vi "benchmark-TagDB.vi"() -> (2 "read":dbl=2.8434400558471685e-05 format="%#_6f", 3 "write":dbl=2.78111743927002e-05 format="%#_6f")   [LabVIEW 2017]
uses:
  a6fc632b-2e92-436d-bf5a-00a40263cc33.vi
  5f513741-77c9-4122-96c3-2ffecd0507aa.vi
  TagDB/_Support/DataAccess/_NameCacher.vi
  TagDB/_Support/DataAccess/_datatypeChecker.vi
  TagDB/_Support/DataAccess/TagDB Ref to DVR.vi
  <vilib>/Utility/Data Type/Get Type Information.vi
  <vilib>/Utility/error.llb/Trim Whitespace.vi
  TagDB/_Support/Error/_[error50000]Invalid DB REF.vi
  TagDB/_Support/Error/_[error50002]Invalid DataType.vi
  <userlib>/_OpenG.lib/md5/md5.llb/MD5 Message Digest (Binary String)__ogtk.vi
  TagDB/TagDB(DEV).lvlib
panel:
  out "write 2":dbl=2.78111743927002e-05 caption="write" format="%#_6f"
  out "length":i32=1170
  out "outside":i32=499
  out "unit (s)":cluster{dbl[]}[](graph)=[{[4.010200500488281e-05, 2.005577087402344e-05, 3.0074119567871094e-05, 3.0078887939453124e-05, 3.0078887939453124e-05, 3.0078887939453124e-05, 2.0051002502441405e-05, 3.0078887939453124e-05, 3.0078887939453124e-05, 3.0078887939453124e-05, 3.0083656311035158e-05, 2.0847320556640624e-05, 2.9277801513671874e-05, 3.0078887939453124e-05, 3.0236244201660155e-05, 3.071784973144531e-05, 2.9430389404296874e-05, 2.002716064453125e-05, 2.9959678649902343e-05, 3.0078887939453124e-05, 3.0074119567871094e-05, 3.0231475830078124e-05, 2.0260810852050782e-05, 2.987384796142578e-05, 2.9926300048828124e-05, 3.0083656311035158e-05, 3.0069351196289064e-05, 3.0231475830078124e-05, 2.005577087402344e-05, 3.0074119567871094e-05, 2.9926300048828124e-05, 3.0078887939453124e-05, 3.0083656311035158e-05, 3.0078887939453124e-05, 2.0046234130859375e-05, 3.0088424682617188e-05, 3.0074119567871094e-05, 3.0078887939453124e-05, 3.0078887939453124e-05, 3.0078887939453124e-05, 2.0051002502441405e-05, 3.0078887939453124e-05, 3.0078887939453124e-05, 3.0078887939453124e-05, 3.0074119567871094e-05, 3.0078887939453124e-05, 2.005577087402344e-05, 3.0083656311035158e-05, 3.0078887939453124e-05, 3.0069351196289064e-05, 3.0083656311035158e-05, 3.0078887939453124e-05, 3.0078887939453124e-05, 2.0046234130859375e-05, 3.0083656311035158e-05, 3.0078887939453124e-05, 3.0078887939453124e-05, 3.0078887939453124e-05, 3.0083656311035158e-05, 2.0046234130859375e-05, 3.0078887939453124e-05, 3.0078887939453124e-05, 3.0083656311035158e-05, 3.0078887939453124e-05, 3.0069351196289064e-05, 2.006053924560547e-05, 3.0078887939453124e-05, 3.0078887939453124e-05, 3.0078887939453124e-05, 3.0074119567871094e-05, 2.005577087402344e-05, 3.0078887939453124e-05, 3.0078887939453124e-05, 3.0074119567871094e-05, 3.0078887939453124e-05, 3.0088424682617188e-05, 2.0046234130859375e-05, 3.0074119567871094e-05, 3.0078887939453124e-05, 3.0078887939453124e-05, 3.0083656311035158e-05, 3.0078887939453124e-05, 2.0046234130859375e-05, 3.0078887939453124e-05, 3.0083656311035158e-05, 3.0078887939453124e-05, 3.0078887939453124e-05, 3.0231475830078124e-05, 2.0051002502441405e-05, 2.9926300048828124e-05, 3.0078887939453124e-05, 3.0078887939453124e-05, 3.0074119567871094e-05, 2.005577087402344e-05, 3.0088424682617188e-05, 3.0074119567871094e-05, 3.0078887939453124e-05, 3.0069351196289064e-05, 2.005577087402344e-05, 3.0083656311035158e-05, 3.0078887939453124e-05, 3.0078887939453124e-05, 3.0074119567871094e-05, 3.0078887939453124e-05, 2.005577087402344e-05, 3.0069351196289064e-05, 3.0088424682617188e-05, 3.0074119567871094e-05, 3.0078887939453124e-05, 3.0078887939453124e-05, 3.0083656311035158e-05, 2.005577087402344e-05, 3.0069351196289064e-05, 3.0078887939453124e-05, 3.0083656311035158e-05, 3.0078887939453124e-05, 3.0078887939453124e-05, 2.0051002502441405e-05, 3.0078887939453124e-05, 3.0078887939453124e-05, 3.0078887939453124e-05, 3.0074119567871094e-05, 3.0078887939453124e-05, 2.005577087402344e-05, 3.0078887939453124e-05, 3.0083656311035158e-05, 3.0069351196289064e-05, 3.0078887939453124e-05, 3.024101257324219e-05, 2.0046234130859375e-05, 2.9931068420410158e-05, 3.0069351196289064e-05, 3.0088424682617188e-05, 3.0074119567871094e-05, 3.0231475830078124e-05, 3.0078887939453124e-05, 2.9931068420410158e-05, 3.0069351196289064e-05, 3.0078887939453124e-05, 2.005577087402344e-05, 2.0203590393066405e-05, 2.9931068420410158e-05, 3.0069351196289064e-05, 3.0083656311035158e-05, 3.0231475830078124e-05, 3.0078887939453124e-05, 2.005577087402344e-05, 2.9921531677246094e-05, 3.0078887939453124e-05, 3.0231475830078124e-05, 3.0078887939453124e-05, 3.0083656311035158e-05, 2.0046234130859375e-05, 2.9926300048828124e-05, 3.0078887939453124e-05, 3.0083656311035158e-05, 3.0069351196289064e-05, 2.02178955078125e-05, 3.0069351196289064e-05, 2.9931068420410158e-05, 3.0078887939453124e-05, 3.0074119567871094e-05, 3.0078887939453124e-05, 2.005577087402344e-05, 3.0078887939453124e-05, 3.0074119567871094e-05, 3.0078887939453124e-05, 3.0078887939453124e-05, 3.0078887939453124e-05, 3.0083656311035158e-05, 2.0046234130859375e-05, 3.0088424682617188e-05, 3.0069351196289064e-05, 3.0083656311035158e-05, 3.0078887939453124e-05, 3.0078887939453124e-05, 3.0074119567871094e-05, 2.005577087402344e-05, 3.0078887939453124e-05, 3.0078887939453124e-05, 3.0074119567871094e-05, 3.0078887939453124e-05, 3.0078887939453124e-05, 3.0078887939453124e-05, 2.005577087402344e-05, 3.0074119567871094e-05, 3.0078887939453124e-05, 3.0078887939453124e-05, 3.0083656311035158e-05, 3.0078887939453124e-05, 2.0046234130859375e-05, 3.0083656311035158e-05, 3.0078887939453124e-05, 3.0078887939453124e-05, 3.0078887939453124e-05, 3.0078887939453124e-05, 2.0051002502441405e-05, 3.0078887939453124e-05, 3.0231475830078124e-05, 3.0078887939453124e-05, 2.9931068420410158e-05, 3.0069351196289064e-05, 2.0847320556640624e-05, 2.944469451904297e-05, 3.0078887939453124e-05, 3.0069351196289064e-05, 2.9935836791992188e-05, 2.0203590393066405e-05, 3.071784973144531e-05, 2.9430389404296874e-05, 3.072261810302735e-05, 2.943992614746094e-05, 3.0078887939453124e-05, 2.005577087402344e-05, 3.0078887939453124e-05, 3.0074119567871094e-05, 3.0078887939453124e-05, 3.0078887939453124e-05, 3.0083656311035158e-05, 2.005577087402344e-05, 3.0069351196289064e-05, 3.072261810302735e-05, 2.943992614746094e-05, 3.0088424682617188e-05, 2.0046234130859375e-05, 3.0074119567871094e-05, 3.0078887939453124e-05, 3.0078887939453124e-05, 3.0078887939453124e-05, 3.0078887939453124e-05, 2.0051002502441405e-05, 3.0078887939453124e-05, 3.0078887939453124e-05, 3.0083656311035158e-05, 3.070831298828125e-05, 2.9449462890625e-05, 3.0078887939453124e-05, 2.0051002502441405e-05, 3.071784973144531e-05, 2.943992614746094e-05, 3.0074119567871094e-05, 3.0078887939453124e-05, 3.070354461669922e-05, 1.9431114196777344e-05, 3.0074119567871094e-05, 3.0078887939453124e-05, 3.0078887939453124e-05, 3.0112266540527343e-05, 3.005027770996094e-05, 2.005577087402344e-05, 3.0069351196289064e-05, 3.0078887939453124e-05, 3.0083656311035158e-05, 3.0078887939453124e-05, 3.0078887939453124e-05, 2.0051002502441405e-05, 3.0078887939453124e-05, 3.0078887939453124e-05, 3.0074119567871094e-05, 3.0083656311035158e-05, 3.0074119567871094e-05, 2.005577087402344e-05, 3.0078887939453124e-05, 3.0074119567871094e-05, 3.0078887939453124e-05, 3.0078887939453124e-05, 3.072261810302735e-05, 1.941680908203125e-05, 3.070831298828125e-05, 2.943992614746094e-05, 3.0083656311035158e-05, 3.0078887939453124e-05, 3.0078887939453124e-05, 2.0046234130859375e-05, 3.0083656311035158e-05, 3.0078887939453124e-05, 3.0078887939453124e-05, 3.0078887939453124e-05, 2.0051002502441405e-05, 3.071784973144531e-05, 2.943992614746094e-05, 3.0078887939453124e-05, 3.0083656311035158e-05, 3.0078887939453124e-05, 2.0046234130859375e-05, 3.0083656311035158e-05, 3.0078887939453124e-05, 3.0069351196289064e-05, 2.9935836791992188e-05, 3.0074119567871094e-05, 3.0078887939453124e-05, 2.0051002502441405e-05, 3.0231475830078124e-05, 3.0078887939453124e-05, 2.9926300048828124e-05, 3.0088424682617188e-05, 3.0074119567871094e-05, 3.0078887939453124e-05, 2.020835876464844e-05, 3.0069351196289064e-05, 2.9931068420410158e-05, 3.0078887939453124e-05, 3.0078887939453124e-05, 3.0074119567871094e-05, 3.0078887939453124e-05, 3.0078887939453124e-05, 2.0051002502441405e-05, 3.0078887939453124e-05, 3.0078887939453124e-05, 3.0078887939453124e-05, 3.0083656311035158e-05, 3.0078887939453124e-05, 3.0069351196289064e-05, 2.005577087402344e-05, 3.0083656311035158e-05, 3.0078887939453124e-05, 3.0078887939453124e-05, 3.0074119567871094e-05, 3.0078887939453124e-05, 2.005577087402344e-05, 3.0078887939453124e-05, 3.0074119567871094e-05, 3.0078887939453124e-05, 3.0078887939453124e-05, 3.0078887939453124e-05, 2.0051002502441405e-05, 3.0078887939453124e-05, 3.024101257324219e-05, 3.0069351196289064e-05, 2.9931068420410158e-05, 2.0046234130859375e-05, 3.024101257324219e-05, 3.0112266540527343e-05, 2.9888153076171875e-05, 3.0112266540527343e-05, 3.0045509338378905e-05, 3.0078887939453124e-05, 2.0051002502441405e-05, 3.0078887939453124e-05, 3.0231475830078124e-05, 3.0078887939453124e-05, 2.9931068420410158e-05, 3.0069351196289064e-05, 2.0847320556640624e-05, 2.943992614746094e-05, 3.072261810302735e-05, 2.9430389404296874e-05, 3.0083656311035158e-05, 3.0078887939453124e-05, 2.005577087402344e-05, 3.0078887939453124e-05, 3.0074119567871094e-05, 2.9935836791992188e-05, 3.0221939086914064e-05, 3.0078887939453124e-05, 2.005577087402344e-05, 3.071308135986328e-05, 2.943992614746094e-05, 3.0112266540527343e-05, 3.005027770996094e-05, 3.071784973144531e-05, 2.943992614746094e-05, 2.0046234130859375e-05, 3.0083656311035158e-05, 2.9926300048828124e-05, 3.0231475830078124e-05, 3.0078887939453124e-05, 2.0051002502441405e-05, 3.0078887939453124e-05, 3.071784973144531e-05, 2.943992614746094e-05, 3.0074119567871094e-05, 3.0078887939453124e-05, 2.0694732666015624e-05, 2.9435157775878905e-05, 3.0078887939453124e-05, 3.0088424682617188e-05, 3.0074119567871094e-05, 3.0078887939453124e-05, 2.0046234130859375e-05, 3.0078887939453124e-05, 3.0083656311035158e-05, 3.0078887939453124e-05, 3.0088424682617188e-05, 2.0046234130859375e-05, 3.0074119567871094e-05, 3.0078887939453124e-05, 3.0078887939453124e-05, 3.0078887939453124e-05, 3.0083656311035158e-05, 2.0046234130859375e-05, 3.0078887939453124e-05, 3.0078887939453124e-05, 3.0074119567871094e-05, 3.0078887939453124e-05, 3.0078887939453124e-05, 2.005577087402344e-05, 3.0083656311035158e-05, 3.0078887939453124e-05, 3.0088424682617188e-05, 3.006458282470703e-05, 3.0078887939453124e-05, 2.005577087402344e-05, 3.0074119567871094e-05, 3.0078887939453124e-05, 3.0078887939453124e-05, 3.0078887939453124e-05, 3.0083656311035158e-05, 3.0078887939453124e-05, 2.0046234130859375e-05, 3.0078887939453124e-05, 3.0083656311035158e-05, 3.0078887939453124e-05, 3.0078887939453124e-05, 3.0074119567871094e-05, 3.0078887939453124e-05, 2.0694732666015624e-05, 2.943992614746094e-05, 3.0078887939453124e-05, 3.0083656311035158e-05, 3.070831298828125e-05, 2.943992614746094e-05, 2.005577087402344e-05, 2.9931068420410158e-05, 3.0069351196289064e-05, 3.0231475830078124e-05, 3.0083656311035158e-05, 3.009319305419922e-05, 3.005504608154297e-05, 1.99127197265625e-05, 3.0226707458496094e-05, 3.0078887939453124e-05, 3.0078887939453124e-05, 3.072261810302735e-05, 2.928733825683594e-05, 2.0046234130859375e-05, 3.0078887939453124e-05, 3.0236244201660155e-05, 3.0069351196289064e-05, 3.025054931640625e-05, 2.9764175415039063e-05, 2.0051002502441405e-05, 3.0069351196289064e-05, 3.0088424682617188e-05, 3.0226707458496094e-05, 3.0078887939453124e-05, 2.9926300048828124e-05, 2.0051002502441405e-05, 3.0078887939453124e-05, 3.0078887939453124e-05, 3.0078887939453124e-05, 3.0231475830078124e-05, 2.9931068420410158e-05, 2.0046234130859375e-05, 3.0078887939453124e-05, 3.0083656311035158e-05, 3.0231475830078124e-05, 2.9926300048828124e-05, 2.0046234130859375e-05, 3.0083656311035158e-05, 3.0078887939453124e-05, 3.0078887939453124e-05, 3.0231475830078124e-05, 2.9921531677246094e-05, 3.0088424682617188e-05, 2.0046234130859375e-05, 3.0074119567871094e-05, 3.0078887939453124e-05, 3.0078887939453124e-05, 3.0078887939453124e-05, 3.0083656311035158e-05, 2.005577087402344e-05, 3.0069351196289064e-05, 3.0083656311035158e-05, 3.0078887939453124e-05, 3.0078887939453124e-05, 3.0078887939453124e-05, 2.0051002502441405e-05, 3.0078887939453124e-05, 3.0231475830078124e-05, 3.0078887939453124e-05, 2.9931068420410158e-05, 3.0078887939453124e-05, 2.0046234130859375e-05, 3.0078887939453124e-05, 3.0231475830078124e-05, 3.0083656311035158e-05, 2.9926300048828124e-05, 3.0074119567871094e-05, 2.0847320556640624e-05, 2.9430389404296874e-05, 2.9926300048828124e-05, 3.0083656311035158e-05, 3.0088424682617188e-05, 3.0069351196289064e-05, 2.0051002502441405e-05, 3.0078887939453124e-05, 3.0078887939453124e-05, 3.0078887939453124e-05, 3.0078887939453124e-05]}, ...(2 in all)]
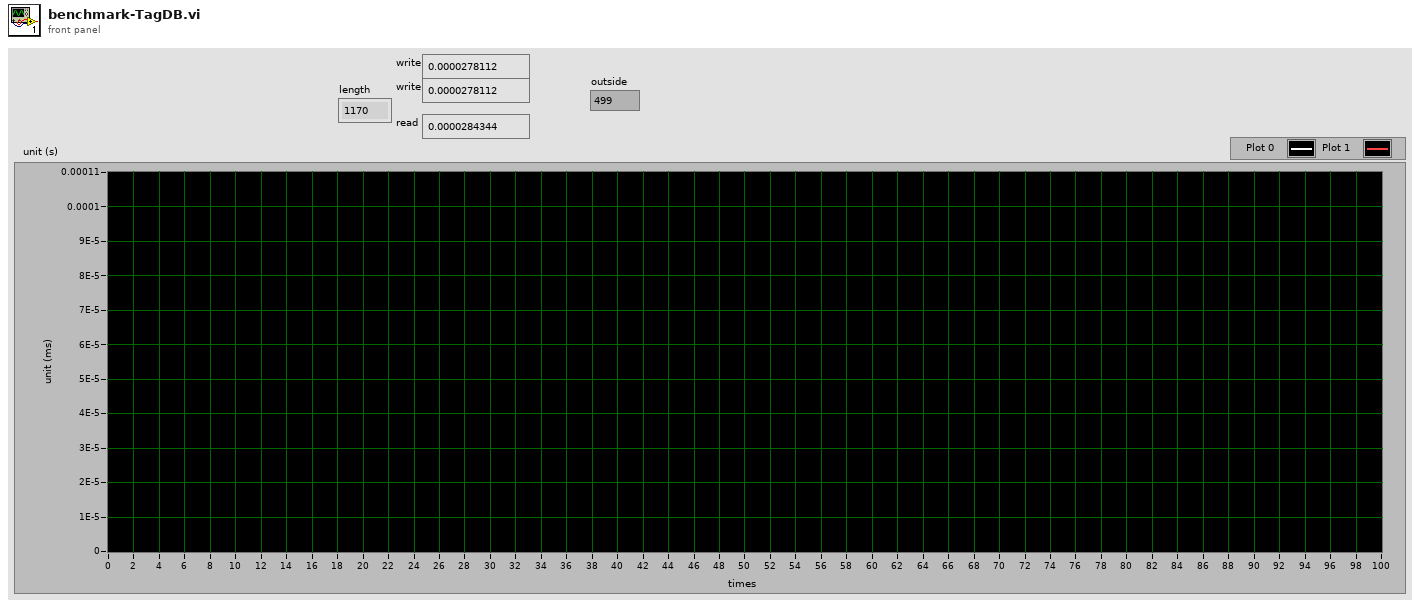
[diagram p1: front panel]
types:
  T1 = cluster{"error constant":errorcluster, "error constant 2":errorcluster, "error constant 3":errorcluster, "error constant 4":errorcluster, "error constant 5":errorcluster, "error constant 6":errorcluster, "error constant 7":errorcluster, "error constant 8":errorcluster, "error constant 9":errorcluster, "error constant 10":errorcluster, "error constant 11":errorcluster, "error constant 12":errorcluster, "error constant 13":errorcluster, "error constant 14":errorcluster, "error constant 15":errorcluster, "error constant 16":errorcluster, "error constant 17":errorcluster, "error constant 18":errorcluster, "error constant 19":errorcluster, "error constant 20":errorcluster, "error constant 21":errorcluster, "error constant 22":errorcluster, "error constant 23":errorcluster, "error constant 24":errorcluster, "error constant 25":errorcluster, "error constant 26":errorcluster, "error constant 27":errorcluster, "error constant 28":errorcluster, "error constant 29":errorcluster, "error constant 30":errorcluster, "error constant 31":errorcluster, "error constant 32":errorcluster, "error constant 33":errorcluster, "error constant 34":errorcluster, "error constant 35":errorcluster, "error constant 36":errorcluster, "error constant 37":errorcluster, "error constant 38":errorcluster, "error constant 39":errorcluster, "error constant 40":errorcluster, "error constant 41":errorcluster, "error constant 42":errorcluster, "error constant 43":errorcluster, "error constant 44":errorcluster, "error constant 45":errorcluster, "error constant 46":errorcluster, "error constant 47":errorcluster, "error constant 48":errorcluster, "error constant 49":errorcluster, "error constant 50":errorcluster, "error constant 51":errorcluster, "error constant 52":errorcluster, "error constant 53":errorcluster, "error constant 54":errorcluster, "error constant 55":errorcluster, "error constant 56":errorcluster, "error constant 57":errorcluster, "error constant 58":errorcluster, "error constant 59":errorcluster, "error constant 60":errorcluster, "error constant 61":errorcluster, "error constant 62":errorcluster, "error constant 63":errorcluster, "error constant 64":errorcluster, "error constant 65":errorcluster, cluster{"error constant":errorcluster, "error constant 2":errorcluster, "error constant 3":errorcluster, "error constant 4":errorcluster, "error constant 5":errorcluster, "error constant 6":errorcluster, "error constant 7":errorcluster, "error constant 8":errorcluster, "error constant 9":errorcluster, "error constant 10":errorcluster, "error constant 11":errorcluster, "error constant 12":errorcluster, "error constant 13":errorcluster, "error constant 14":errorcluster, "error constant 15":errorcluster, "error constant 16":errorcluster, "error constant 17":errorcluster, "error constant 18":errorcluster, "error constant 19":errorcluster, "error constant 20":errorcluster, "error constant 21":errorcluster, "error constant 22":errorcluster, "error constant 23":errorcluster, "error constant 24":errorcluster, "error constant 25":errorcluster, "error constant 26":errorcluster, "error constant 27":errorcluster, "error constant 28":errorcluster, "error constant 29":errorcluster, "error constant 30":errorcluster, "error constant 31":errorcluster, "error constant 32":errorcluster, "error constant 33":errorcluster, "error constant 34":errorcluster, "error constant 35":errorcluster, "error constant 36":errorcluster, "error constant 37":errorcluster, "error constant 38":errorcluster, "error constant 39":errorcluster, "error constant 40":errorcluster, "error constant 41":errorcluster, "error constant 42":errorcluster, "error constant 43":errorcluster, "error constant 44":errorcluster, "error constant 45":errorcluster, "error constant 46":errorcluster, "error constant 47":errorcluster, "error constant 48":errorcluster, "error constant 49":errorcluster, "error constant 50":errorcluster, "error constant 51":errorcluster, "error constant 52":errorcluster, "error constant 53":errorcluster, "error constant 54":errorcluster, "error constant 55":errorcluster, "error constant 56":errorcluster, "error constant 57":errorcluster, "error constant 58":errorcluster, "error constant 59":errorcluster, "error constant 60":errorcluster, "error constant 61":errorcluster, "error constant 62":errorcluster, "error constant 63":errorcluster, "error constant 64":errorcluster, "error constant 65":errorcluster}}
  T2 = typedef "TagDB(DEV).lvlib/TagContainer.ctl" = refnum<k1>
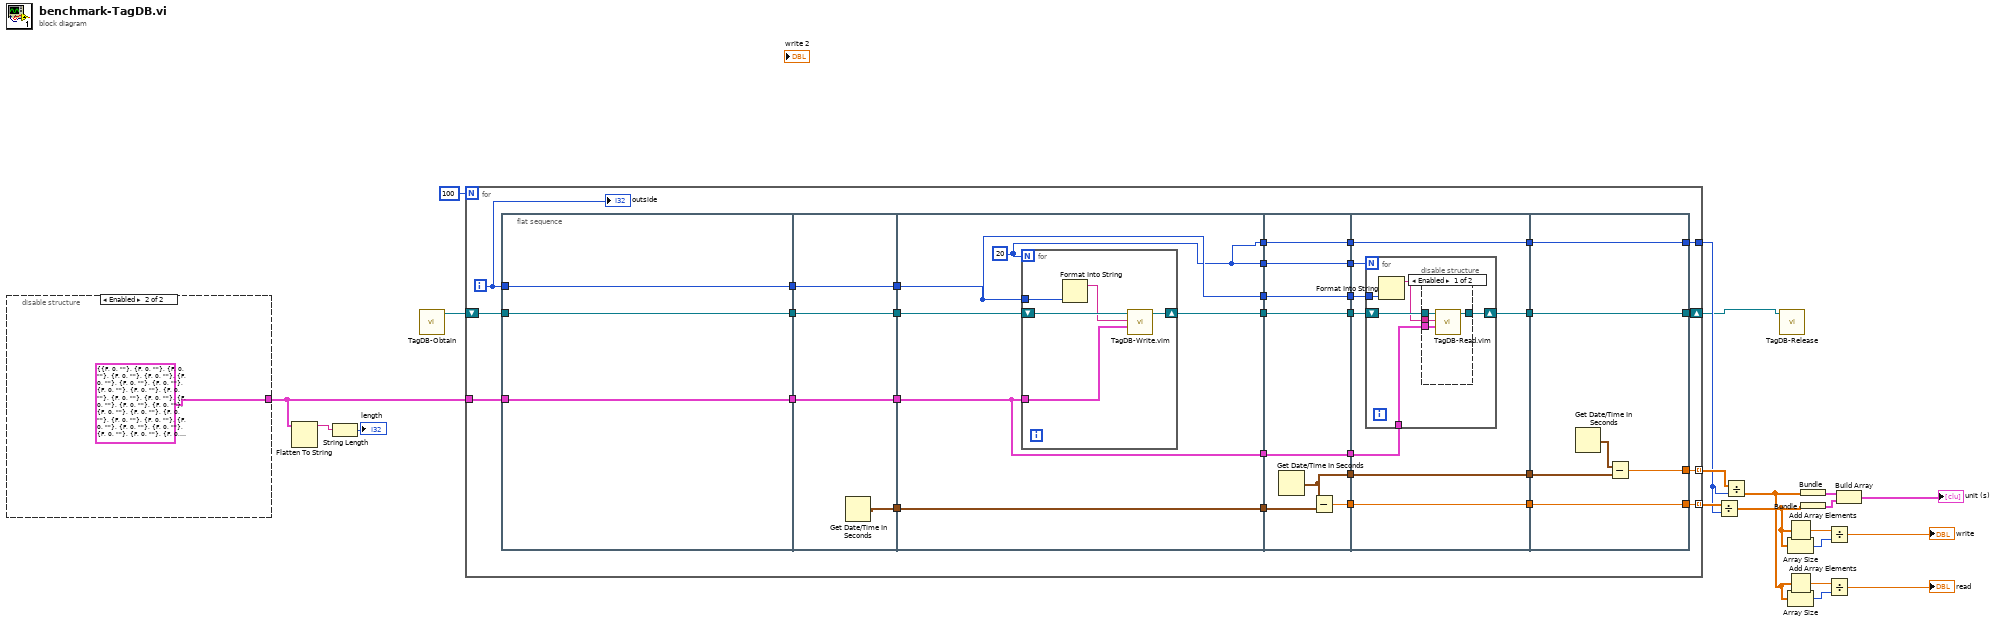
[diagram p0: block diagram]
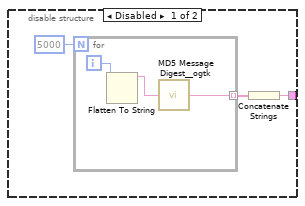
[diagram p2: hidden frame]
diagram:
  n1 = disable-structure shown="Enabled" {
    disable-tunnel: [w21 T1 {"error constant"={"status"=FALSE, "code"=0, "source"=""}, "error constant 2"={"status"=FALSE, "code"=0, "source"=""}, "error constant 3"={"status"=FALSE, "code"=0, "source"=""}, "error constant 4"={"status"=FALSE, "code"=0, "source"=""}, "error constant 5"={"status"=FALSE, "code"=0, "source"=""}, "error constant 6"={"status"=FALSE, "code"=0, "source"=""}, "error constant 7"={"status"=FALSE, "code"=0, "source"=""}, "error constant 8"={"status"=FALSE, "code"=0, "source"=""}, "error constant 9"={"status"=FALSE, "code"=0, "source"=""}, "error constant 10"={"status"=FALSE, "code"=0, "source"=""}, "error constant 11"={"status"=FALSE, "code"=0, "source"=""}, "error constant 12"={"status"=FALSE, "code"=0, "source"=""}, "error constant 13"={"status"=FALSE, "code"=0, "source"=""}, "error constant 14"={"status"=FALSE, "code"=0, "source"=""}, "error constant 15"={"status"=FALSE, "code"=0, "source"=""}, "error constant 16"={"status"=FALSE, "code"=0, "source"=""}, "error constant 17"={"status"=FALSE, "code"=0, "source"=""}, "error constant 18"={"status"=FALSE, "code"=0, "source"=""}, "error constant 19"={"status"=FALSE, "code"=0, "source"=""}, "error constant 20"={"status"=FALSE, "code"=0, "source"=""}, "error constant 21"={"status"=FALSE, "code"=0, "source"=""}, "error constant 22"={"status"=FALSE, "code"=0, "source"=""}, "error constant 23"={"status"=FALSE, "code"=0, "source"=""}, "error constant 24"={"status"=FALSE, "code"=0, "source"=""}, "error constant 25"={"status"=FALSE, "code"=0, "source"=""}, "error constant 26"={"status"=FALSE, "code"=0, "source"=""}, "error constant 27"={"status"=FALSE, "code"=0, "source"=""}, "error constant 28"={"status"=FALSE, "code"=0, "source"=""}, "error constant 29"={"status"=FALSE, "code"=0, "source"=""}, "error constant 30"={"status"=FALSE, "code"=0, "source"=""}, "error constant 31"={"status"=FALSE, "code"=0, "source"=""}, "error constant 32"={"status"=FALSE, "code"=0, "source"=""}, "error constant 33"={"status"=FALSE, "code"=0, "source"=""}, "error constant 34"={"status"=FALSE, "code"=0, "source"=""}, "error constant 35"={"status"=FALSE, "code"=0, "source"=""}, "error constant 36"={"status"=FALSE, "code"=0, "source"=""}, "error constant 37"={"status"=FALSE, "code"=0, "source"=""}, "error constant 38"={"status"=FALSE, "code"=0, "source"=""}, "error constant 39"={"status"=FALSE, "code"=0, "source"=""}, "error constant 40"={"status"=FALSE, "code"=0, "source"=""}, "error constant 41"={"status"=FALSE, "code"=0, "source"=""}, "error constant 42"={"status"=FALSE, "code"=0, "source"=""}, "error constant 43"={"status"=FALSE, "code"=0, "source"=""}, "error constant 44"={"status"=FALSE, "code"=0, "source"=""}, "error constant 45"={"status"=FALSE, "code"=0, "source"=""}, "error constant 46"={"status"=FALSE, "code"=0, "source"=""}, "error constant 47"={"status"=FALSE, "code"=0, "source"=""}, "error constant 48"={"status"=FALSE, "code"=0, "source"=""}, "error constant 49"={"status"=FALSE, "code"=0, "source"=""}, "error constant 50"={"status"=FALSE, "code"=0, "source"=""}, "error constant 51"={"status"=FALSE, "code"=0, "source"=""}, "error constant 52"={"status"=FALSE, "code"=0, "source"=""}, "error constant 53"={"status"=FALSE, "code"=0, "source"=""}, "error constant 54"={"status"=FALSE, "code"=0, "source"=""}, "error constant 55"={"status"=FALSE, "code"=0, "source"=""}, "error constant 56"={"status"=FALSE, "code"=0, "source"=""}, "error constant 57"={"status"=FALSE, "code"=0, "source"=""}, "error constant 58"={"status"=FALSE, "code"=0, "source"=""}, "error constant 59"={"status"=FALSE, "code"=0, "source"=""}, "error constant 60"={"status"=FALSE, "code"=0, "source"=""}, "error constant 61"={"status"=FALSE, "code"=0, "source"=""}, "error constant 62"={"status"=FALSE, "code"=0, "source"=""}, "error constant 63"={"status"=FALSE, "code"=0, "source"=""}, "error constant 64"={"status"=FALSE, "code"=0, "source"=""}, "error constant 65"={"status"=FALSE, "code"=0, "source"=""}, {"error constant"={"status"=FALSE, "code"=0, "source"=""}, "error constant 2"={"status"=FALSE, "code"=0, "source"=""}, "error constant 3"={"status"=FALSE, "code"=0, "source"=""}, "error constant 4"={"status"=FALSE, "code"=0, "source"=""}, "error constant 5"={"status"=FALSE, "code"=0, "source"=""}, "error constant 6"={"status"=FALSE, "code"=0, "source"=""}, "error constant 7"={"status"=FALSE, "code"=0, "source"=""}, "error constant 8"={"status"=FALSE, "code"=0, "source"=""}, "error constant 9"={"status"=FALSE, "code"=0, "source"=""}, "error constant 10"={"status"=FALSE, "code"=0, "source"=""}, "error constant 11"={"status"=FALSE, "code"=0, "source"=""}, "error constant 12"={"status"=FALSE, "code"=0, "source"=""}, "error constant 13"={"status"=FALSE, "code"=0, "source"=""}, "error constant 14"={"status"=FALSE, "code"=0, "source"=""}, "error constant 15"={"status"=FALSE, "code"=0, "source"=""}, "error constant 16"={"status"=FALSE, "code"=0, "source"=""}, "error constant 17"={"status"=FALSE, "code"=0, "source"=""}, "error constant 18"={"status"=FALSE, "code"=0, "source"=""}, "error constant 19"={"status"=FALSE, "code"=0, "source"=""}, "error constant 20"={"status"=FALSE, "code"=0, "source"=""}, "error constant 21"={"status"=FALSE, "code"=0, "source"=""}, "error constant 22"={"status"=FALSE, "code"=0, "source"=""}, "error constant 23"={"status"=FALSE, "code"=0, "source"=""}, "error constant 24"={"status"=FALSE, "code"=0, "source"=""}, "error constant 25"={"status"=FALSE, "code"=0, "source"=""}, "error constant 26"={"status"=FALSE, "code"=0, "source"=""}, "error constant 27"={"status"=FALSE, "code"=0, "source"=""}, "error constant 28"={"status"=FALSE, "code"=0, "source"=""}, "error constant 29"={"status"=FALSE, "code"=0, "source"=""}, "error constant 30"={"status"=FALSE, "code"=0, "source"=""}, "error constant 31"={"status"=FALSE, "code"=0, "source"=""}, "error constant 32"={"status"=FALSE, "code"=0, "source"=""}, "error constant 33"={"status"=FALSE, "code"=0, "source"=""}, "error constant 34"={"status"=FALSE, "code"=0, "source"=""}, "error constant 35"={"status"=FALSE, "code"=0, "source"=""}, "error constant 36"={"status"=FALSE, "code"=0, "source"=""}, "error constant 37"={"status"=FALSE, "code"=0, "source"=""}, "error constant 38"={"status"=FALSE, "code"=0, "source"=""}, "error constant 39"={"status"=FALSE, "code"=0, "source"=""}, "error constant 40"={"status"=FALSE, "code"=0, "source"=""}, "error constant 41"={"status"=FALSE, "code"=0, "source"=""}, "error constant 42"={"status"=FALSE, "code"=0, "source"=""}, "error constant 43"={"status"=FALSE, "code"=0, "source"=""}, "error constant 44"={"status"=FALSE, "code"=0, "source"=""}, "error constant 45"={"status"=FALSE, "code"=0, "source"=""}, "error constant 46"={"status"=FALSE, "code"=0, "source"=""}, "error constant 47"={"status"=FALSE, "code"=0, "source"=""}, "error constant 48"={"status"=FALSE, "code"=0, "source"=""}, "error constant 49"={"status"=FALSE, "code"=0, "source"=""}, "error constant 50"={"status"=FALSE, "code"=0, "source"=""}, "error constant 51"={"status"=FALSE, "code"=0, "source"=""}, "error constant 52"={"status"=FALSE, "code"=0, "source"=""}, "error constant 53"={"status"=FALSE, "code"=0, "source"=""}, "error constant 54"={"status"=FALSE, "code"=0, "source"=""}, "error constant 55"={"status"=FALSE, "code"=0, "source"=""}, "error constant 56"={"status"=FALSE, "code"=0, "source"=""}, "error constant 57"={"status"=FALSE, "code"=0, "source"=""}, "error constant 58"={"status"=FALSE, "code"=0, "source"=""}, "error constant 59"={"status"=FALSE, "code"=0, "source"=""}, "error constant 60"={"status"=FALSE, "code"=0, "source"=""}, "error constant 61"={"status"=FALSE, "code"=0, "source"=""}, "error constant 62"={"status"=FALSE, "code"=0, "source"=""}, "error constant 63"={"status"=FALSE, "code"=0, "source"=""}, "error constant 64"={"status"=FALSE, "code"=0, "source"=""}, "error constant 65"={"status"=FALSE, "code"=0, "source"=""}}}] -> w17
    frame Disabled {
      n2 = for {
        N: 5000 -> [_]
        tunnel: [w26] -> w23 mode=indexing
        i -> [w25]
        n3 = Flatten To String(anything=w25) -> (data string=w24:string)  [unwired: 3 in, 2 out]
        n4 = call-poly <userlib>:"MD5 Message Digest__ogtk.vi"("Message"=w24) -> ("MD5 Message Digest"=w26:string)
      }
      n5 = Concatenate Strings(w23) -> (w21:string)
    }
    frame Enabled {
    }
  }
  n6 = Flatten To String(anything=w17) -> (data string=w16:string)  [unwired: 3 in, 2 out]
  n7 = String Length(string=w16) -> (length=→"length":i32)
  n8 = call "TagDB-Obtain.vi"() -> ("TagContainer"=w2:T2)  [unwired: 5 in, 2 out]
  n9 = for {
    N: 100 -> [_]
    tunnel: [w56] -> w20 mode=indexing
    tunnel: [w55] -> w3
    tunnel: w17 -> [w42]
    shift-right: [w40] -> w1
    shift-left: w2 -> [w41]
    tunnel: [w35] -> w4 mode=indexing
    i -> [w53]
    n10 = flat-sequence {
      tunnel: w53 -> [w61]
      tunnel: [w59] -> w47
      tunnel: [w60] -> w45
      tunnel: [w61] -> w44
      tunnel: w42 -> [w60]
      tunnel: w41 -> [w59]
      tunnel: [w65] -> w58
      tunnel: [w64] -> w48
      tunnel: w47 -> [w64]
      tunnel: [w63] -> w46
      tunnel: w45 -> [w63]
      tunnel: w44 -> [w62]
      tunnel: [w62] -> w43
      tunnel: w58 -> [w71]
      tunnel: [w71] -> w57
      tunnel: [w67] -> w54
      tunnel: [w69] -> w49
      tunnel: w48 -> [w70]
      tunnel: w46 -> [w66]
      tunnel: w43 -> [w68]
      tunnel: [w67] -> w33
      tunnel: [w68] -> w30
      tunnel: [w66] -> w29
      tunnel: w57 -> [w81]
      tunnel: w54 -> [w83]
      tunnel: [w84] -> w52
      tunnel: [w83] -> w51
      tunnel: [w82] -> w50
      tunnel: w49 -> [w82]
      tunnel: [w77] -> w37
      tunnel: w33 -> [w80]
      tunnel: [w80] -> w32
      tunnel: [w79] -> w31
      tunnel: w30 -> [w79]
      tunnel: w29 -> [w78]
      tunnel: [w78] -> w28
      tunnel: w52 -> [w92]
      tunnel: w51 -> [w91]
      tunnel: w50 -> [w89]
      tunnel: [w92] -> w39
      tunnel: [w91] -> w38
      tunnel: w37 -> [w90]
      tunnel: [w90] -> w36
      tunnel: [w88] -> w34
      tunnel: w32 -> [w87]
      tunnel: w31 -> [w86]
      tunnel: w28 -> [w85]
      tunnel: [w106] -> w40
      tunnel: [w107] -> w55
      tunnel: [w108] -> w56
      tunnel: w39 -> [w108]
      tunnel: w38 -> [w107]
      tunnel: w36 -> [w104]
      tunnel: [w103] -> w35
      tunnel: w34 -> [w106]
      frame #0 {
      }
      frame #1 {
        n11 = Get Date/Time In Seconds() -> (seconds since 1Jan1904=w65:timestamp)
      }
      frame #2 {
        w67 = 20
        n12 = for {
          N: w67 -> [_]
          tunnel: w66 -> [w73]
          tunnel: w68 -> [w76]
          shift-right: [w74] -> w69
          shift-left: w70 -> [w75]
          n13 = Format Into String(w76) -> (resulting string=w72:string)  [unwired: 3 in, 1 out]
          n14 = call "TagDB-Write.vim"("Value"=w73, "name"=w72, "TagContainer"=w75) -> ("TagContainer(dup)"=w74:T2)  [unwired: 6 in, 2 out]
        }
      }
      frame #3 {
        n15 = Get Date/Time In Seconds() -> (seconds since 1Jan1904=w77:timestamp)
        n16 = Subtract(x=w77, y=w81) -> (x-y=w84:dbl)
      }
      frame #4 {
        n17 = for {
          N: w87 -> [_]
          shift-right: [w96] -> w88
          shift-left: w89 -> [w95]
          tunnel: w86 -> [w97]
          tunnel: w85 -> [w93]
          n18 = Format Into String(w97) -> (resulting string=w94:string)  [unwired: 3 in, 1 out]
          n19 = disable-structure shown="Enabled" {
            disable-tunnel: [w101 w102] -> w96
            disable-tunnel: w95 -> [w100 w102]
            disable-tunnel: w94 -> [w99 _]
            disable-tunnel: w93 -> [w98 _]
            frame Enabled {
              n20 = call "TagDB-Read.vim"("Type"=w98, "name"=w99, "TagContainer"=w100) -> ("TagContainer(dup)"=w101:T2)  [unwired: 3 in, 5 out]
            }
            frame Disabled {
            }
          }
        }
      }
      frame #5 {
        n21 = Get Date/Time In Seconds() -> (seconds since 1Jan1904=w105:timestamp)
        n22 = Subtract(x=w105, y=w104) -> (x-y=w103:dbl)
      }
    }
    "outside" <- w53
  }
  n23 = Divide(x=w20, y=w3) -> (x/y=w12:dbl[])
  n24 = Divide(x=w4, y=w3) -> (x/y=w5:dbl[])
  n25 = call "TagDB-Release.vi"("TagContainer"=w1) -> ()  [unwired: 10 in, 1 out]
  n26 = Add Array Elements(numeric array=w12) -> (sum=w14:dbl)
  n27 = Array Size(array=w12) -> (size(s)=w13:i32)
  n28 = Add Array Elements(numeric array=w5) -> (sum=w7:dbl)
  n29 = Array Size(array=w5) -> (size(s)=w8:i32)
  n30 = Bundle(w5) -> (w11:cluster{dbl[]})  [unwired: 1 in]
  n31 = Bundle(w12) -> (w10:cluster{dbl[]})  [unwired: 1 in]
  n32 = Divide(x=w14, y=w13) -> (x/y=→"write":dbl)
  n33 = Divide(x=w7, y=w8) -> (x/y=→"read":dbl)
  n34 = Build Array(w11, w10) -> (→"unit (s)":cluster{dbl[]}[])
